vi "Read Slot Programming Modes Supported.vi"(8 "error in (no error)":errorcluster, 11 "9233 in":refnum<class "9233.lvclass">) -> (0 "error out":errorcluster, 2 "Slot Programming Modes Supported":u8, 3 "9233 out":refnum<class "9233.lvclass">)   [LabVIEW 2017, in "Modules.lvlib" / "9233.lvclass"]
uses:
  9233.lvclass
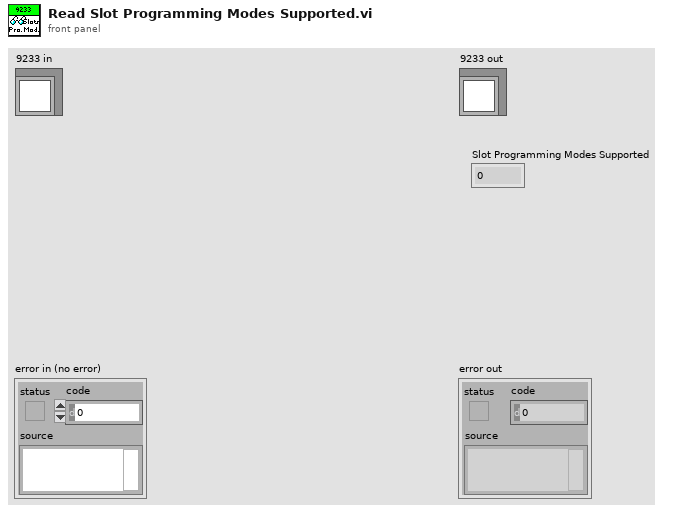
[diagram p1: front panel]
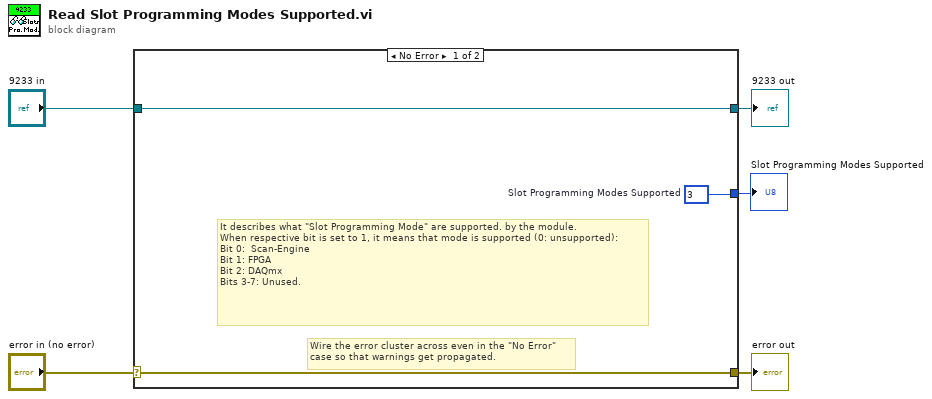
[diagram p0: block diagram]
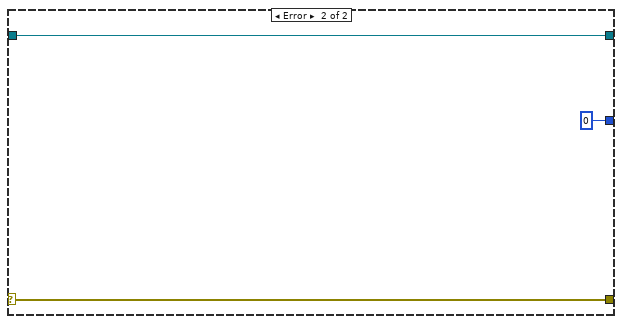
[diagram p2: hidden frame]
diagram:
  n1 = case shown="No Error" "error in (no error)" {
    selector: "error in (no error)" -> [w8 w11]
    tunnel: [w8 w11] -> w4
    tunnel: [w7 w10] -> w2
    tunnel: "9233 in" -> [w7 w10]
    tunnel: [w6 u8 0 ("Slot Programming Modes Supported")] -> w1
    frame No Error {
      w6 = u8 3  # Slot Programming Modes Supported
      # "It describes what \"Slot Programming Mode\" are supported. by the module.\nWhen respective bit is set to 1, it means that mode is supported (0: unsupported):\nBit 0:  Scan-Engine\nBit 1: FPGA\nBit 2: DAQmx\nBits 3-7: Unused."
      # "Wire the error cluster across even in the \"No Error\"\ncase so that warnings get propagated."
    }
    frame Error {
    }
  }
  "error out" <- w4
  "9233 out" <- w2
  "Slot Programming Modes Supported" <- w1
